vi "Engine Out - DI Firing Order.vi"(0 "Injector 1":T1, 1 "Injector 2":T1, 2 "Injector 3":T1, 3 "Injector 4":T1, 4 "Injector 5":T1, 5 "Injector 6":T1, 7 "Injector 7":T1, 9 "Injector 8":T1) -> (11 "DI4-2":T1, 13 "DI4-1":T1, 14 "DI1-1":T1, 15 "DI1-2":T1, 16 "DI2-1":T1, 17 "DI2-2":T1, 18 "DI3-1":T1, 19 "DI3-2":T1)   [LabVIEW 2015, in "ECS-RT.lvlib"]
uses:
  ECS-RT.lvlib
  Typedefs/Raw Outputs/DI.ctl
  Globals/TDC Globals.vi
  ECS-Shared.lvlib
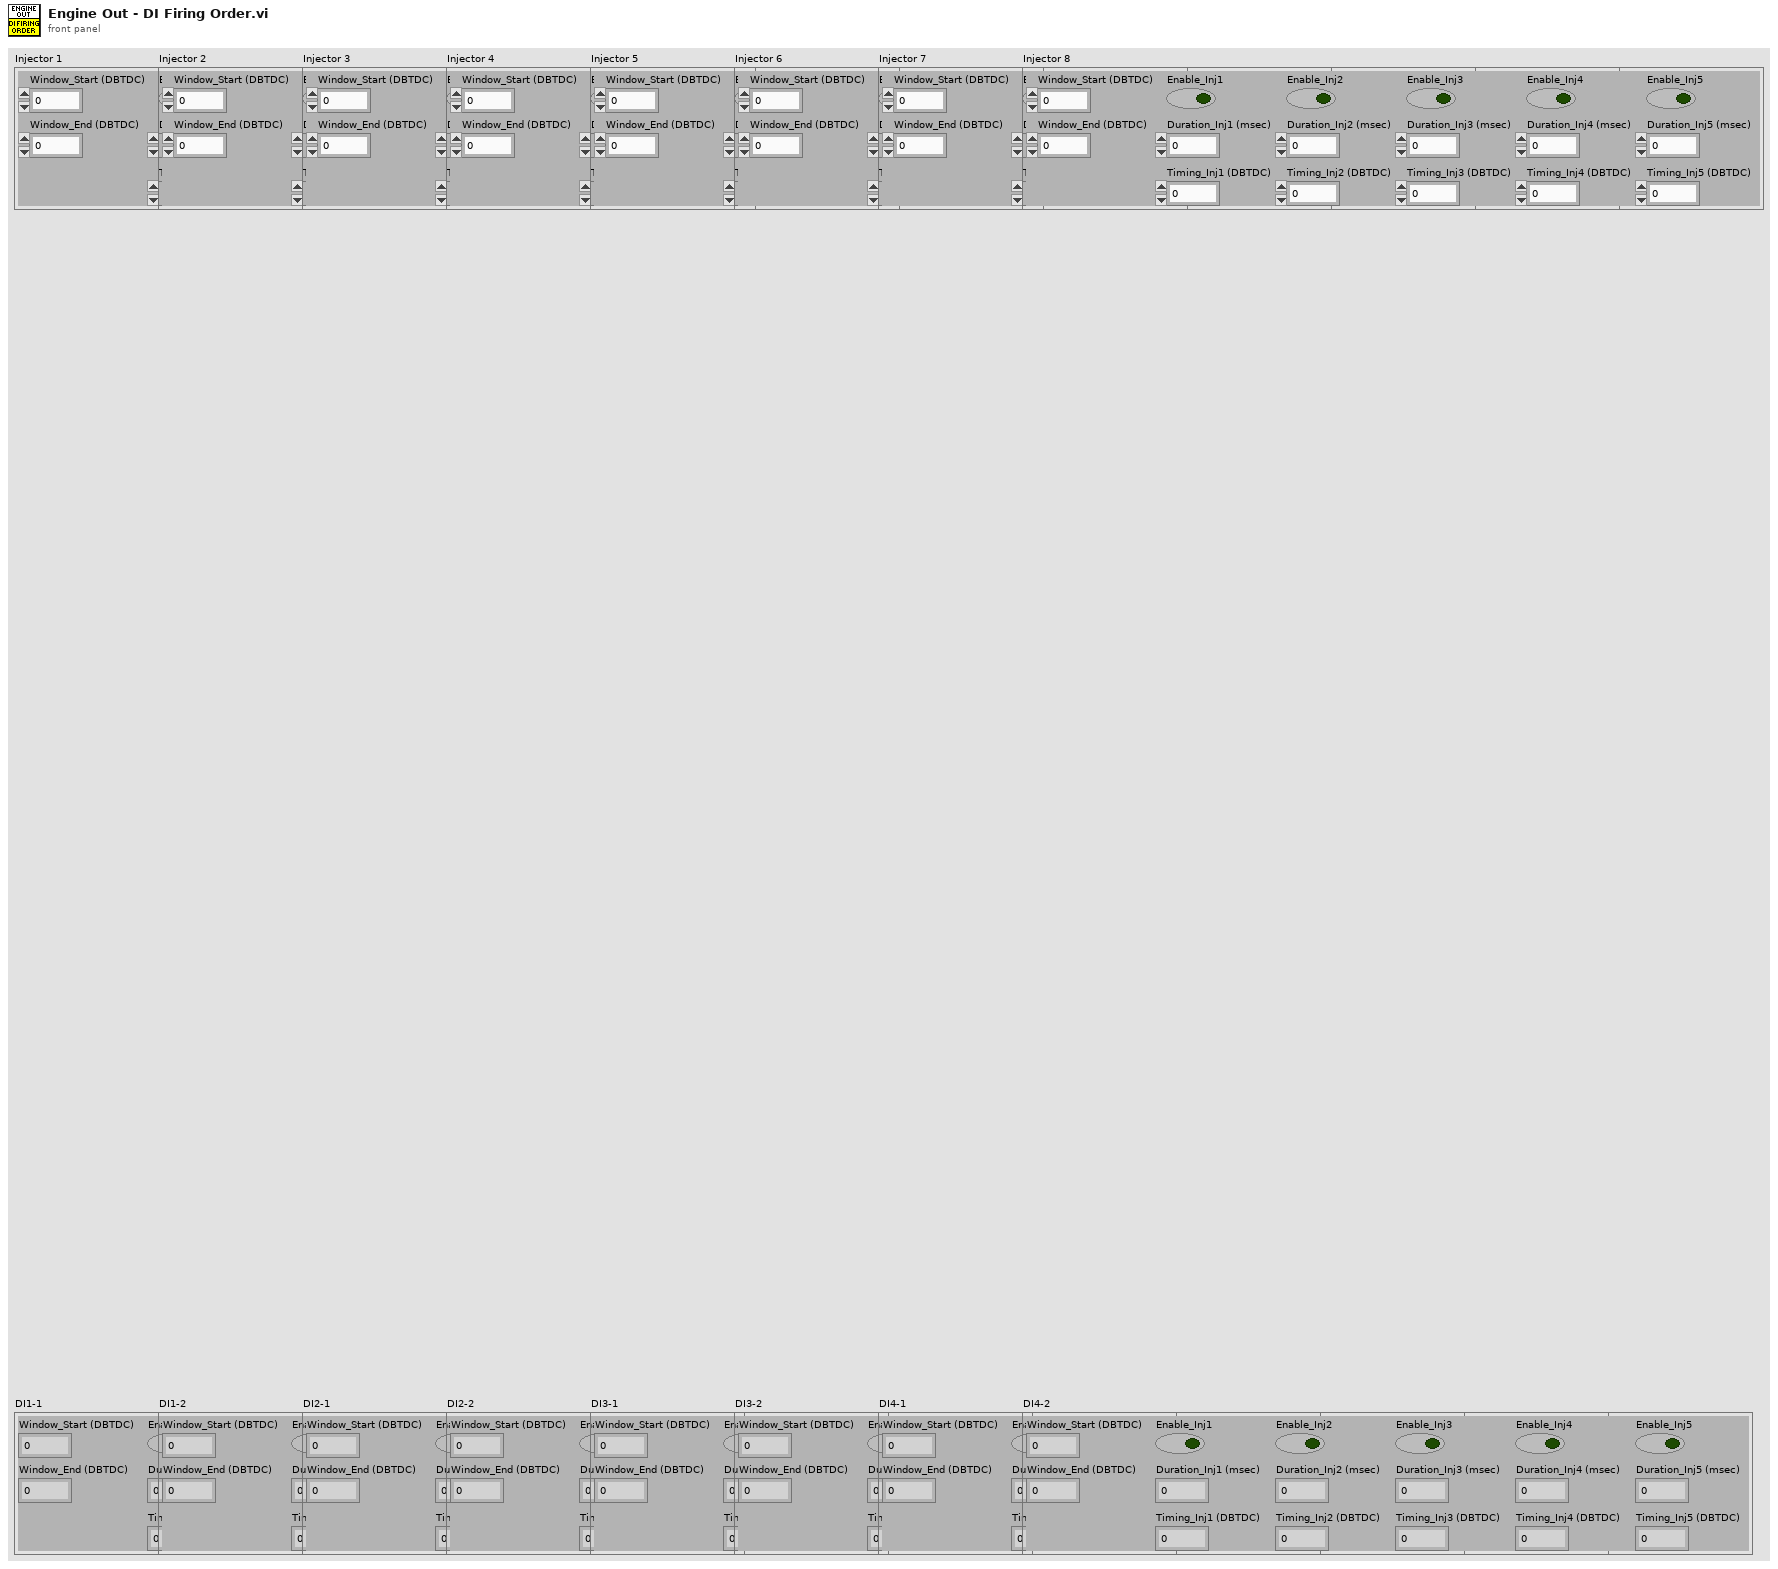
[diagram p1: front panel]
types:
  T1 = typedef "ECS-Shared.lvlib/DI.ctl" = cluster{"Window_Start (DBTDC)":sgl, "Window_End (DBTDC)":sgl, "Enable_Inj1":bool, "Duration_Inj1 (msec)":sgl, "Timing_Inj1 (DBTDC)":sgl, "Enable_Inj2":bool, "Duration_Inj2 (msec)":sgl, "Timing_Inj2 (DBTDC)":sgl, "Enable_Inj3":bool, "Duration_Inj3 (msec)":sgl, "Timing_Inj3 (DBTDC)":sgl, "Enable_Inj4":bool, "Duration_Inj4 (msec)":sgl, "Timing_Inj4 (DBTDC)":sgl, "Enable_Inj5":bool, "Duration_Inj5 (msec)":sgl, "Timing_Inj5 (DBTDC)":sgl}
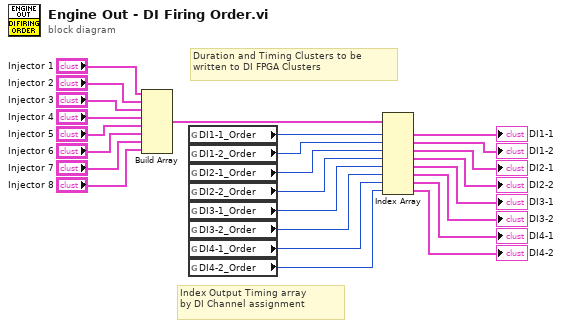
[diagram p0: block diagram]
diagram:
  # "Duration and Timing Clusters to be written to DI FPGA Clusters"
  # "Index Output Timing array\nby DI Channel assignment"
  n1 = Build Array("Injector 1", "Injector 2", "Injector 3", "Injector 4", "Injector 5", "Injector 6", "Injector 7", "Injector 8") -> (w9:T1[])
  n2 = global read "TDC Globals.vi" "DI1-1_Order"() -> (w18:i32)
  n3 = global read "TDC Globals.vi" "DI1-2_Order"() -> (w19:i32)
  n4 = global read "TDC Globals.vi" "DI2-1_Order"() -> (w20:i32)
  n5 = global read "TDC Globals.vi" "DI2-2_Order"() -> (w21:i32)
  n6 = global read "TDC Globals.vi" "DI3-1_Order"() -> (w22:i32)
  n7 = global read "TDC Globals.vi" "DI3-2_Order"() -> (w23:i32)
  n8 = global read "TDC Globals.vi" "DI4-1_Order"() -> (w24:i32)
  n9 = global read "TDC Globals.vi" "DI4-2_Order"() -> (w25:i32)
  n10 = Index Array(array=w9, index #1=w18, index #2=w19, index #3=w20, index #4=w21, index #5=w22, index #6=w23, index #7=w24, index #8=w25) -> (element #1=→"DI1-1":T1, element #2=→"DI1-2":T1, element #3=→"DI2-1":T1, element #4=→"DI2-2":T1, element #5=→"DI3-1":T1, element #6=→"DI3-2":T1, element #7=→"DI4-1":T1, element #8=→"DI4-2":T1)
